vi "PathPlanner_PathFinder_InitializeWorkerThread.vi"   [LabVIEW 2019, in "PathPlanner24.lvlib"]
uses:
  PathPlanner24.lvlib
  PathPlanner_PathFinder_Globals.vi
  PathPlanner_PathFinder_WorkerThread.vi
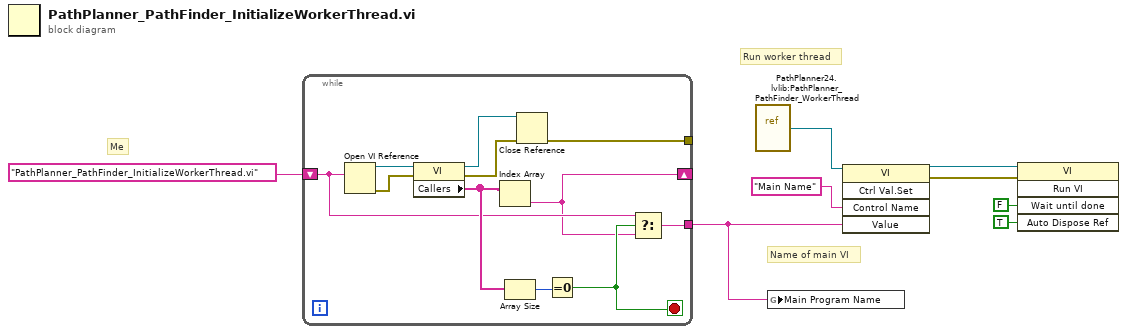
[diagram p0: block diagram]
diagram:
  # "Me"
  # "Name of main VI"
  # "Run worker thread"
  n1 = while {
    shift-right: [w13] -> _
    shift-left: "PathPlanner_PathFinder_InitializeWorkerThread.vi" -> [w14]
    tunnel: [w12] -> w1
    tunnel: [w9] -> _
    stop <- w15 stop-if-true
    n2 = Open VI Reference(vi path=w14) -> (vi reference=w19:refnum<vi>, error out=w11:errorcluster)  [unwired: 5 in]
    n3 = property class="VI"(reference=w19, error in=w11) -> (reference out=w18:refnum<vi>, error out=w10:errorcluster, "Callers"=w17:string[])
    n4 = Index Array(array=w17) -> (element=w13:string)  [unwired: 1 in]
    n5 = Array Size(array=w17) -> (size(s)=w16:i32)
    n6 = Close Reference(reference=w18, error in (no error)=w10) -> (error out=w9:errorcluster)
    n7 = Equal To 0?(x=w16) -> (x = 0?=w15:bool)
    n8 = Select(t=w14, s=w15, f=w13) -> (s? t:f=w12:string)
  }
  n9 = vi-ref "PathPlanner24.lvlib:PathPlanner_PathFinder_WorkerThread.vi"() -> (w7:refnum<vi>)
  n10 = global write "PathPlanner_PathFinder_Globals.vi" "Main Program Name"(w1) -> ()
  n11 = invoke class="VI" method="Ctrl Val.Set"(reference=w7, "Control Name"="Main Name", "Value"=w1) -> (reference out=w6:refnum<vi>, error out=w5:errorcluster)  [unwired: 2 in, 3 out]
  n12 = invoke class="VI" method="Run VI"(reference=w6, error in=w5, "Wait until done"=FALSE ("Wait Until Done"), "Auto Dispose Ref"=TRUE ("Auto Dispose Reference")) -> ()  [unwired: 1 in, 5 out]
